vi "Tests.vi"() -> ()   [LabVIEW 2024]
uses:
  <vilib>/DAQmx/create/channels.llb/DAQmx Create Channel (AI-Voltage-Basic).vi
  <vilib>/DAQmx/read.llb/DAQmx Read (Analog DBL 1Chan 1Samp).vi
panel:
  out "data 4":dbl format="%0.2f"
  out "data 3":dbl[](array[numeric]) format="%0.2f"
  out "data 2":dbl
  out "data":dynamicdata(graph)
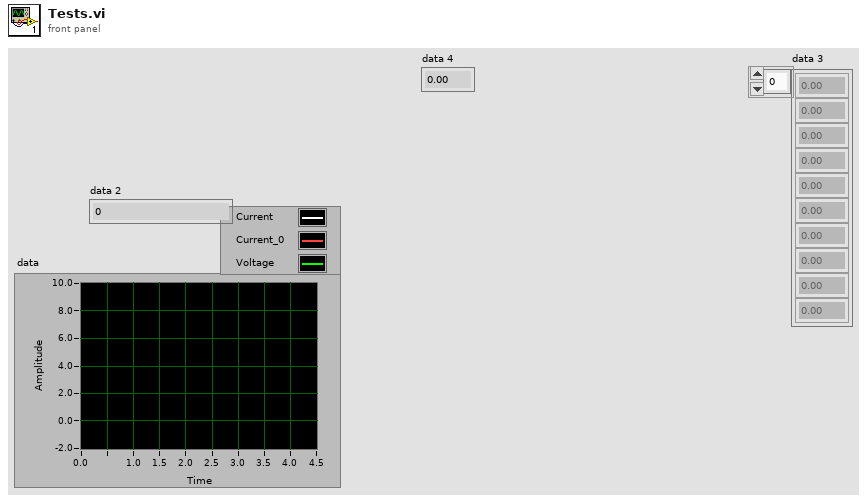
[diagram p1: front panel]
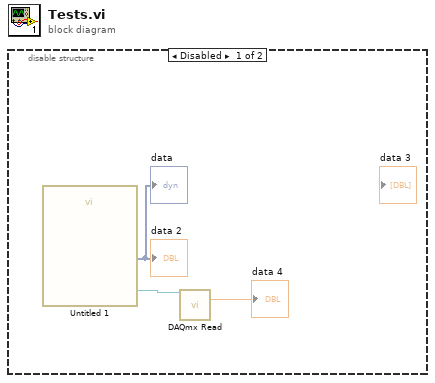
[diagram p0: block diagram]
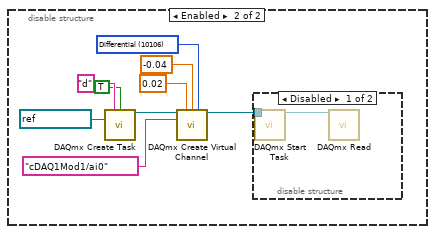
[diagram p2: hidden frame]
diagram:
  n1 = disable-structure shown="Disabled" {
    frame Disabled {
      n2 = call "Untitled 1.vi"() -> ("task out"=w2:refnum<k21>, "data"=→"data" →"data 2":dynamicdata)  [unwired: 17 in, 1 out]
      n3 = call-poly <vilib>:"DAQmx Read.vi"("task/channels in"=w2) -> ("data"=→"data 4":dbl)  [unwired: 12 in, 2 out]
    }
    frame Enabled {
      w6 = 10106 items=["Default"=-1, "RSE"=10083, "NRSE"=10078, "Differential"=10106, "Pseudodifferential"=12529] ("input terminal configuration")
      n4 = call <vilib>:"DAQmx Create Task.vi"("new task name"="d", "auto cleanup"=TRUE, "task to copy"=refnum<k21> "TaskTest" ("task in")) -> ("task out"=w9:refnum<k21>)  [unwired: 11 in, 1 out]
      n5 = call-poly <vilib>:"DAQmx Create Virtual Channel.vi"("task in"=w9, "maximum value"=0.02, "minimum value"=-0.04, "input terminal configuration"=w6, "physical channels"=tag "cDAQ1Mod1/ai0") -> ("task out"=w12:refnum<k21>)  [unwired: 9 in, 1 out]
      n6 = disable-structure shown="Disabled" {
        disable-tunnel: w12 -> [w14 _]
        frame Disabled {
          n7 = call <vilib>:"DAQmx Start Task.vi"("task/channels in"=w14) -> ("task out"=w13:refnum<k21>)  [unwired: 13 in, 1 out]
          n8 = call-poly <vilib>:"DAQmx Read.vi"("task/channels in"=w13) -> ()  [unwired: 12 in, 3 out]
        }
        frame Enabled {
        }
      }
    }
  }
